vi "Merge Diff Images.vi"(8 "ID":i32, 9 "Before = F | After = T?":bool, 10 "Diff PNG Files":path[](array[path])) -> ()   [LabVIEW 2020, in "Graphical Diff.lvlib"]
uses:
  Graphical Diff.lvlib
  4bd7a358-025b-436a-b08a-e2c5914ece35.vi
  6fabf7ea-5db0-41f0-8f7d-caee261b24fd.vi
  <vilib>/numeric/Random Number (Range) I64.vi
  <vilib>/numeric/sub_Random U32.vi
  <vilib>/Comparison/Equal/Equal Functor/Equal Functor.lvclass
panel:
  out "colors":u32[](array[colorbox])
  out "clean picture":picture
  out "size(s)":i32[](array[numeric])
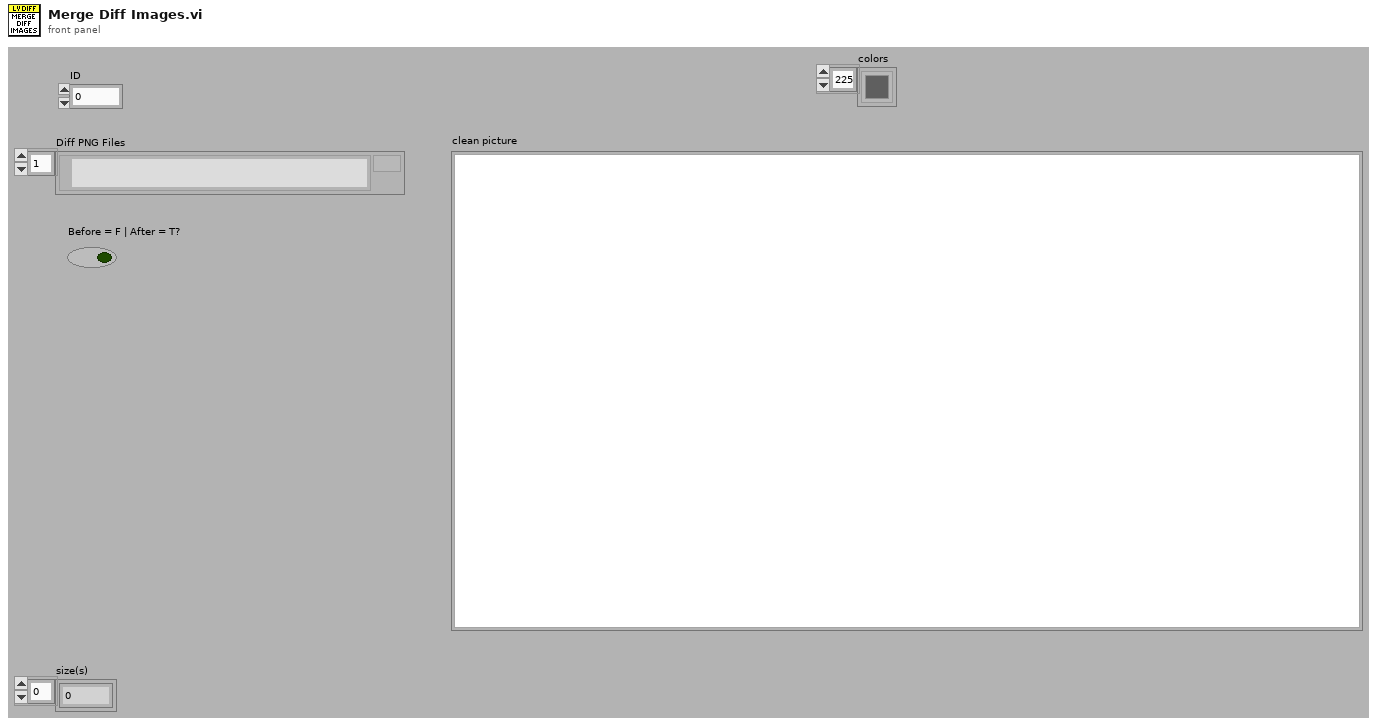
[diagram p1: front panel]
types:
  T1 = typedef "imagedata.ctl" = cluster{"image type":i32, "image depth":i32, "image":u8[], "mask":u8[], "colors":u32[], "Rectangle":cluster{"left":i16, "top":i16, "right":i16, "bottom":i16}}
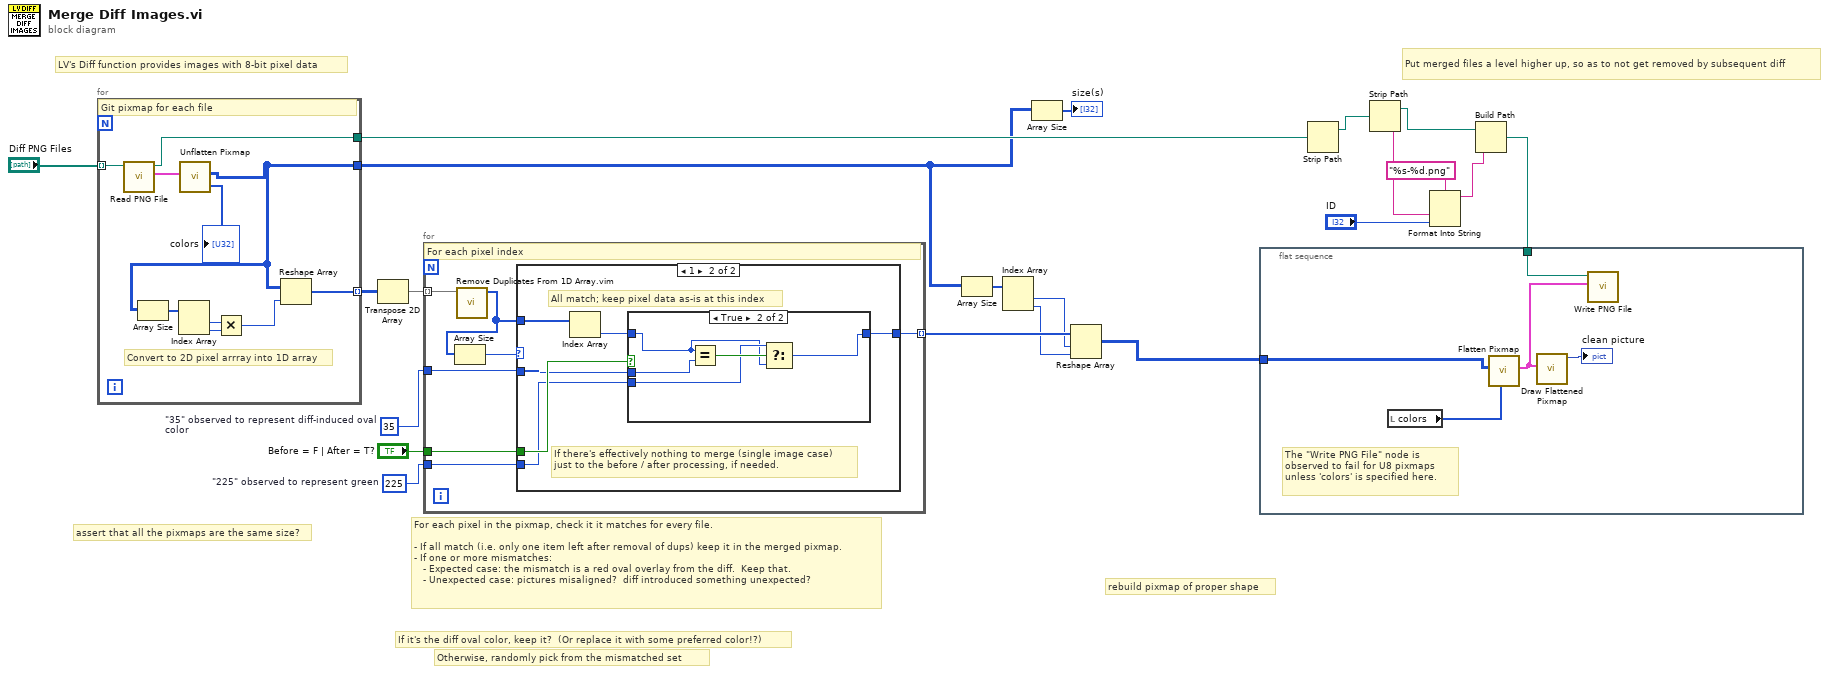
[diagram p0: block diagram]
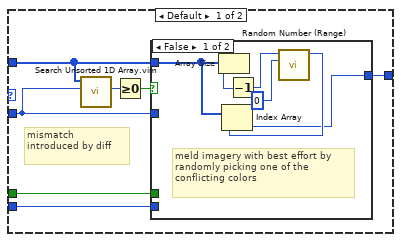
[diagram p2: hidden frame]
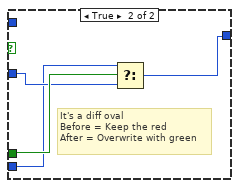
[diagram p3: hidden frame]
diagram:
  w5 = u8 225  # "225" observed to represent green
  w6 = u8 35  # "35" observed to represent diff-induced oval color
  # "Put merged files a level higher up, so as to not get removed by subsequent diff"
  # "If it's the diff oval color, keep it?  (Or replace it with some preferred color!?)"
  # "Otherwise, randomly pick from the mismatched set"
  # "LV's Diff function provides images with 8-bit pixel data"
  # "rebuild pixmap of proper shape"
  # "assert that all the pixmaps are the same size?"
  # "For each pixel in the pixmap, check it it matches for every file.\n\n- If all match (i.e. only one item left after removal of dups) keep it in the merged pixmap.\n- If one or more mismatches:\n   - Expected case: the mismatch is a red oval overlay from the diff.  Keep that.\n   - Unexpected case: pictures misaligned?  diff introduced something unexpected?"
  n1 = for {
    tunnel: [w23] -> w13
    tunnel: [w30] -> w20
    tunnel: "Diff PNG Files" -> [w29] mode=indexing
    tunnel: [w28] -> w17 mode=indexing
    # "Convert to 2D pixel arrray into 1D array"
    # "Git pixmap for each file"
    n2 = call <vilib>:"Read PNG File.vi"("path to PNG file"=w29) -> ("image data"=w31:T1, "path"=w30:path)  [unwired: 8 in, 1 out]
    n3 = call <vilib>:"Unflatten Pixmap.vi"("image data"=w31) -> ("8-bit pixmap"=w23:u8[][], "colors"=→"colors":u32[])  [unwired: 4 in, 5 out]
    n4 = Array Size(array=w23) -> (size(s)=w27:i32[])
    n5 = Index Array(array=w27) -> (element #1=w25:i32, element #2=w26:i32)  [unwired: 2 in]
    n6 = Multiply(x=w25, y=w26) -> (x*y=w24:i32)
    n7 = Reshape Array(w23, w24) -> (w28:u8[])
  }
  n8 = Transpose 2D Array(2D array=w17) -> (transposed array=w16:u8[][])
  n9 = for {
    tunnel: w16 -> [w38] mode=indexing
    tunnel: [w35] -> w15 mode=indexing
    tunnel: "Before = F | After = T?" -> [w34]
    tunnel: w6 -> [w33]
    tunnel: w5 -> [w32]
    # "For each pixel index"
    n10 = call "Remove Duplicates From 1D Array.vim"("array"=w38) -> ("array with duplicates removed"=w36:u8[])  [unwired: 10 in]
    n11 = Array Size(array=w36) -> (size(s)=w37:i32)
    n12 = case shown="1" w37 {
      tunnel: w36 -> [w44 w61]
      tunnel: [w45 w59] -> w35
      tunnel: w34 -> [w41 w60]
      tunnel: w33 -> [w40 w57]
      tunnel: w32 -> [w39 w56]
      frame Default {
        # "mismatch introduced by diff"
        n13 = call "Search Unsorted 1D Array.vim"("element"=w40, "unsorted 1D array"=w44) -> ("index of element"=w43:i32)  [unwired: 9 in]
        n14 = Greater Or Equal To 0?(x=w43) -> (x >= 0?=w42:bool)
        n15 = case shown="False" w42 {
          tunnel: [w49 w53] -> w45
          tunnel: w44 -> [w46 _]
          tunnel: w40 -> [_ w54]
          tunnel: w41 -> [_ w55]
          tunnel: w39 -> [_ w52]
          frame False {
            # "meld imagery with best effort by randomly picking one of the conflicting colors"
            n16 = Array Size(array=w46) -> (size(s)=w51:i32)
            n17 = Decrement(x=w51) -> (x-1=w48:i32)
            n18 = call-poly <vilib>:"Random Number (Range).vi"("lower bound (-100)"=i64 0, "upper bound (100)"=w48) -> ("number"=w50:i64)  [unwired: 9 in]
            n19 = Index Array(array=w46, index=w50) -> (element=w49:u8)
          }
          frame True {
            # "It's a diff oval\nBefore = Keep the red\nAfter = Overwrite with green"
            n20 = Select(t=w52, s=w55, f=w54) -> (s? t:f=w53:u8)
          }
        }
      }
      frame 1 {
        # "If there's effectively nothing to merge (single image case)\njust to the before / after processing, if needed."
        # "All match; keep pixel data as-is at this index"
        n21 = Index Array(array=w61) -> (element=w58:u8)  [unwired: 1 in]
        n22 = case shown="True" w60 {
          tunnel: [w62 w63] -> w59
          tunnel: w58 -> [w62 w64]
          tunnel: w57 -> [_ w67]
          tunnel: w56 -> [_ w65]
          frame False {
          }
          frame True {
            n23 = Equal?(x=w64, y=w67) -> (x = y?=w66:bool)
            n24 = Select(t=w65, s=w66, f=w64) -> (s? t:f=w63:u8)
          }
        }
      }
    }
  }
  n25 = Array Size(array=w13) -> (size(s)=w14:i32[])
  n26 = Index Array(array=w14) -> (element #1=w12:i32, element #2=w11:i32)  [unwired: 2 in]
  n27 = Array Size(array=w13) -> (size(s)=→"size(s)":i32[])
  n28 = Reshape Array(w15, w12, w11) -> (w10:u8[][])
  n29 = flat-sequence {
    tunnel: w19 -> [w70]
    tunnel: w10 -> [w69]
    frame #0 {
      # "The \"Write PNG File\" node is observed to fail for U8 pixmaps unless 'colors' is specified here."
      n30 = local read "colors"() -> (w68:u32[])
      n31 = call <vilib>:"Flatten Pixmap.vi"("colors"=w68, "8-bit pixmap"=w69) -> ("image data"=w71:T1)  [unwired: 9 in]
      n32 = call <vilib>:"Draw Flattened Pixmap.vi"("image data"=w71) -> ("new picture"=→"clean picture":picture)  [unwired: 8 in]
      n33 = call <vilib>:"Write PNG File.vi"("image data"=w71, "path to PNG file"=w70) -> ()  [unwired: 8 in, 2 out]
    }
  }
  n34 = Strip Path(path=w20) -> (stripped path=w8:path)  [unwired: 1 out]
  n35 = Strip Path(path=w8) -> (stripped path=w7:path, name=w3:string)
  n36 = Format Into String(format string="%s-%d.png", w3, "ID") -> (resulting string=w1:string)  [unwired: 2 in, 1 out]
  n37 = Build Path(base path=w7, name or relative path=w1) -> (appended path=w19:path)
